vi "scan -- update freq PID .vi"() -> ()   [LabVIEW 2010]
uses:
  next chunk read-write PID -- action.ctl
  cursor window action.ctl
  find peak action.ctl
  omega map parameters.ctl
  single fit parameters.ctl
  wavepacket.ctl
  complex region.ctl
  circle corners.ctl
  lorentzian.ctl
  filter method control.ctl
panel:
  in  "file path":path=path "E:/data/Ultrasound/Experiment/ProbeTest/Probe10/YBCO_5/sweep5/June_2012/062112/61.63300K_1500_3500_001_062112.bin"
  out "Plot: All":cluster{"all rows":dbl[], "all rows":dbl[]}[](graph)
  out "Plot: complex plane - filter":cluster{dbl[], dbl[]}[](graph)=[{array[1330 elements], array[1330 elements]}, {array[1329 elements], array[1329 elements]}, {[0.0005479834959150251, 0.000546953765247259, 0.0005438686371204671, 0.000538740287125905, 0.0005315889545180808, 0.0005224428623396648, 0.0005113381060380328, 0.0004983185110130269, 0.00048343545965812373, 0.00046674768857760156, 0.0004483210567799979, 0.0004282282857626905, 0.00040654867251337085, 0.0003833677765610607, 0.00035877708231174, 0.0003328736380011912, 0.00030575967268995, 0.0002775421928119073, 0.0002483325598688017, 0.00021824605093724735, 0.00018740140372277897, 0.00015592034795637287, 0.0001239271249828129, 9.154799743686254e-05, 5.8910750942329136e-05, 2.6144189800587135e-05, -6.622371341154751e-06, -3.925961783568815e-05, -7.163874538163862e-05, -0.00010363196835519849, -0.00013511302412160458, -0.00016595767133607297, -0.00019604418026762728, -0.00022525381321073304, -0.0002534712930887757, -0.00028058525840001674, -0.0003064887027105656, -0.0003310793969598863, -0.00035426029291219646, -0.00037593990616151615, -0.0003960326771788234, -0.0004144593089764271, -0.0004311470800569493, -0.0004460301314118525, -0.00045904972643685837, -0.0004701544827384903, -0.0004793005749169064, -0.00048645190752473054, -0.0004915802575192927, -0.0004946653856460845, -0.0004956951163138507, -0.0004946653856460845, -0.0004915802575192927, -0.00048645190752473054, -0.0004793005749169064, -0.0004701544827384903, -0.00045904972643685826, -0.00044603013141185247, -0.00043114708005694924, -0.00041445930897642707, -0.00039603267717882337, -0.000375939906161516, -0.0003542602929121964, -0.00033107939695988626, -0.0003064887027105655, -0.00028058525840001685, -0.0002534712930887754, -0.00022525381321073293, -0.00019604418026762698, -0.00016595767133607288, -0.00013511302412160458, -0.00010363196835519827, -7.163874538163853e-05, -3.9259617835687814e-05, -6.622371341154649e-06, 2.6144189800587125e-05, 5.891075094232935e-05, 9.154799743686252e-05, 0.00012392712498281324, 0.00015592034795637298, 0.00018740140372277883, 0.00021824605093724757, 0.0002483325598688017, 0.0002775421928119076, 0.0003057596726899501, 0.0003328736380011915, 0.00035877708231174017, 0.0003833677765610607, 0.000406548672513371, 0.0004282282857626906, 0.0004483210567799981, 0.0004667476885776017, 0.00048343545965812373, 0.000498318511013027, 0.0005113381060380328, 0.0005224428623396649, 0.0005315889545180809, 0.000538740287125905, 0.0005438686371204671, 0.000546953765247259], [7.058823573779542e-05, 0.00010335479687953737, 0.00013599204337407076, 0.00016837117092002117, 0.0002003643938935811, 0.00023184544965998714, 0.0002626900968744556, 0.0002927766058060099, 0.00032198623874911566, 0.0003502037186271582, 0.00037731768393839946, 0.0004032211282489483, 0.000427811822498269, 0.0004509927184505791, 0.0004726723316998987, 0.0004927651027172061, 0.0005111917345148098, 0.000527879505595332, 0.0005427625569502352, 0.000555782151975241, 0.0005668869082768729, 0.000576033000455289, 0.0005831843330631132, 0.0005883126830576753, 0.0005913978111844672, 0.0005924275418522333, 0.0005913978111844672, 0.0005883126830576753, 0.0005831843330631132, 0.000576033000455289, 0.0005668869082768729, 0.000555782151975241, 0.0005427625569502351, 0.0005278795055953319, 0.0005111917345148097, 0.0004927651027172061, 0.0004726723316998987, 0.00045099271845057897, 0.0004278118224982689, 0.0004032211282489482, 0.00037731768393839946, 0.0003502037186271582, 0.00032198623874911555, 0.00029277660580600976, 0.0002626900968744555, 0.00023184544965998698, 0.00020036439389358113, 0.00016837117092002114, 0.00013599204337407065, 0.00010335479687953725, 7.058823573779526e-05, 3.7821674596053486e-05, 5.184428101520091e-06, -2.719469944443039e-05, -5.9187922417990366e-05, -9.066897818439646e-05, -0.00012151362539886495, -0.00015160013433041905, -0.00018080976727352478, -0.00020902724715156744, -0.0002361412124628087, -0.0002620446567733575, -0.0002866353510226781, -0.0003098162469749882, -0.0003314958602243079, -0.0003515886312416152, -0.0003700152630392191, -0.00038670303411974106, -0.0004015860854746444, -0.0004146056804996502, -0.00042571043680128214, -0.0004348565289796983, -0.00044200786158752237, -0.00044713621158208453, -0.00045022133970887637, -0.0004512510703766425, -0.00045022133970887637, -0.00044713621158208453, -0.00044200786158752237, -0.0004348565289796982, -0.00042571043680128214, -0.0004146056804996501, -0.0004015860854746443, -0.00038670303411974096, -0.0003700152630392189, -0.0003515886312416151, -0.0003314958602243078, -0.0003098162469749882, -0.00028663535102267787, -0.0002620446567733574, -0.00023614121246280827, -0.00020902724715156717, -0.00018080976727352478, -0.0001516001343304188, -0.00012151362539886471, -9.066897818439597e-05, -5.9187922417990095e-05, -2.719469944443035e-05, 5.184428101520362e-06, 3.782167459605353e-05]}, {array[664 elements], array[664 elements]}, {[0.00034068734716914955, 2.614418980058722e-05, 0.00036184737334241687], [0.00010448980708328159, 7.058823573779542e-05, 0.00015148623079228184]}, {[0.000403257657435818, 0.00040294817556057327, 0.00040263869368532856, 0.00040232921181008384, 0.0004020197299348392, 0.00040171024805959446, 0.00040140076618434974, 0.000401091284309105, 0.0004007818024338603, 0.0004004723205586156, 0.00040016283868337093, 0.0003998533568081262, 0.0003995438749328815, 0.0003992343930576368, 0.00039892491118239206, 0.00039861542930714734, 0.00039830594743190263, 0.00039799646555665797, 0.00039768698368141325, 0.00039737750180616853], [6.852122448113725e-05, 7.270377946499367e-05, 7.688633444885008e-05, 8.10688894327065e-05, 8.525144441656292e-05, 8.943399940041934e-05, 9.361655438427574e-05, 9.779910936813216e-05, 0.00010198166435198858, 0.00010616421933584499, 0.0001103467743197014, 0.00011452932930355783, 0.00011871188428741423, 0.00012289443927127064, 0.00012707699425512707, 0.00013125954923898347, 0.00013544210422283988, 0.0001396246592066963, 0.00014380721419055272, 0.00014798976917440912]}, {[2.614418980058722e-05, 2.875338633115941e-05, 3.13625828617316e-05, 3.397177939230379e-05, 3.658097592287598e-05, 3.9190172453448165e-05, 4.179936898402036e-05, 4.440856551459255e-05, 4.701776204516474e-05, 4.962695857573692e-05, 5.2236155106309116e-05, 5.484535163688131e-05, 5.7454548167453496e-05, 6.006374469802568e-05, 6.267294122859788e-05, 6.528213775917007e-05, 6.789133428974225e-05, 7.050053082031444e-05, 7.310972735088663e-05, 7.571892388145883e-05], [7.058823573779542e-05, 7.058823573779542e-05, 7.058823573779542e-05, 7.058823573779542e-05, 7.058823573779542e-05, 7.058823573779542e-05, 7.058823573779542e-05, 7.058823573779542e-05, 7.058823573779542e-05, 7.058823573779542e-05, 7.058823573779542e-05, 7.058823573779542e-05, 7.058823573779542e-05, 7.058823573779542e-05, 7.058823573779542e-05, 7.058823573779542e-05, 7.058823573779542e-05, 7.058823573779542e-05, 7.058823573779542e-05, 7.058823573779542e-05]}]
  out "Plot: fragment filter":cluster{dbl[], dbl[]}[](graph)
  in  "filter method":T1=enum."three"
  in  "smart filter: span 2":dbl(slide)=0.3493 min=0.0001 max=0.5 step=0.0001 scale=0.0001..0.5 scale format="%#_2g"
  out "lorentzian":T2={"Amplitude"=5.854807827548728e-05, "omega(0)"=3052.344293191275, "Gamma"=0.1436186235030105, "phase"=-1.3766021697880535, "Q"=21253.12315869183, "Norm  Ampl"=0.06539080765156977, "z (inf)"=0.4544427884804473+0.08017129776839105i, "4corners"={"z (-pi/2)"=0.09555591315300638-0.4544427884804473i, "z(inf)"=0.4544427884804473+0.08017129776839105i, "z (pi/2)"=-0.08017129776839105+0.43905817309583195i, "z center"=0.007692307692307665-0.007692307692307665i, "z(0)"=-0.43905817309583195-0.09555591315300638i, "radius"=0.4553086922616207}} {"z (inf)" format="%#9_9f"; "Q" format="%#9_9f"; "phase" format="%#9_9f"; "Gamma" format="%#9_9f"; "omega(0)" format="%#9_9f"}
  out "complex region":T4={"max re"=1.5, "min re"=-1.5, "max im"=1.5, "min im"=-1.5, "delta re"=3.0, "delta im"=3.0, "center re"=0.0, "delta  z"=3.0+3.0i, "center im"=0.0, "center z"=0.0+0.0i, "d im"=0.0, "d re"=0.0, "d z"=0.0+0.0i}
  in  "parameters: wavepacket":T5={"R"=0.5, "wave number"=24.764705882352942, "delta k"=8.0, "radii vector"=[-1.5, -1.4846153846153847, -1.4692307692307693, -1.4538461538461538, -1.4384615384615385, -1.4230769230769231, -1.4076923076923076, -1.3923076923076922, -1.376923076923077, -1.3615384615384616, -1.3461538461538463, -1.3307692307692307, -1.3153846153846154, -1.3, -1.2846153846153845, -1.2692307692307692, -1.2538461538461538, -1.2384615384615385, -1.2230769230769232, -1.2076923076923076, -1.1923076923076923, -1.176923076923077, -1.1615384615384614, -1.146153846153846, -1.1307692307692307, -1.1153846153846154, -1.1, -1.0846153846153845, -1.0692307692307692, -1.0538461538461539, -1.0384615384615383, -1.023076923076923, -1.0076923076923077, -0.9923076923076923, -0.9769230769230769, -0.9615384615384615, -0.9461538461538461, -0.9307692307692308, -0.9153846153846154, -0.8999999999999999, -0.8846153846153846, -0.8692307692307693, -0.8538461538461538, -0.8384615384615384, -0.823076923076923, -0.8076923076923077, -0.7923076923076923, -0.7769230769230768, -0.7615384615384615, -0.7461538461538462, -0.7307692307692307, -0.7153846153846153, -0.7, -0.6846153846153846, -0.6692307692307692, -0.6538461538461537, -0.6384615384615384, -0.6230769230769231, -0.6076923076923076, -0.5923076923076922, -0.5769230769230769, -0.5615384615384615, -0.5461538461538461, -0.5307692307692307, -0.5153846153846153, -0.5, -0.48461538461538467, -0.4692307692307691, -0.4538461538461538, -0.43846153846153846, -0.4230769230769229, -0.4076923076923076, -0.39230769230769225, -0.3769230769230769, -0.3615384615384616, -0.34615384615384603, -0.3307692307692307, -0.3153846153846154, -0.2999999999999998, -0.2846153846153845, -0.26923076923076916, -0.25384615384615383, -0.2384615384615385, -0.22307692307692295, -0.20769230769230762, -0.1923076923076923, -0.17692307692307674, -0.1615384615384614, -0.14615384615384608, -0.13076923076923075, -0.11538461538461542, -0.09999999999999987, -0.08461538461538454, -0.0692307692307692, -0.053846153846153655, -0.038461538461538325, -0.023076923076922995, -0.007692307692307665, 0.007692307692307665, 0.023076923076923217, 0.03846153846153855, 0.05384615384615388, 0.06923076923076943, 0.08461538461538476, 0.10000000000000009, 0.11538461538461542, 0.13076923076923075, 0.1461538461538463, 0.16153846153846163, 0.17692307692307696, 0.1923076923076925, 0.20769230769230784, 0.22307692307692317, 0.2384615384615385, 0.25384615384615383, 0.2692307692307694, 0.2846153846153847, 0.30000000000000004, 0.3153846153846156, 0.3307692307692309, 0.34615384615384626, 0.3615384615384616, 0.3769230769230769, 0.39230769230769247, 0.4076923076923078, 0.42307692307692313, 0.4384615384615387, 0.453846153846154, 0.46923076923076934, 0.48461538461538467, 0.5, 0.5153846153846153, 0.5307692307692307, 0.5461538461538464, 0.5615384615384618, 0.5769230769230771, 0.5923076923076924, 0.6076923076923078, 0.6230769230769231, 0.6384615384615384, 0.6538461538461542, 0.6692307692307695, 0.6846153846153848, 0.7000000000000002, 0.7153846153846155, 0.7307692307692308, 0.7461538461538462, 0.7615384615384615, 0.7769230769230768, 0.7923076923076926, 0.8076923076923079, 0.8230769230769233, 0.8384615384615386, 0.8538461538461539, 0.8692307692307693, 0.8846153846153846, 0.9000000000000004, 0.9153846153846157, 0.930769230769231, 0.9461538461538463, 0.9615384615384617, 0.976923076923077, 0.9923076923076923, 1.0076923076923077, 1.023076923076923, 1.0384615384615388, 1.053846153846154, 1.0692307692307694, 1.0846153846153848, 1.1, 1.1153846153846154, 1.1307692307692307, 1.1461538461538465, 1.1615384615384619, 1.1769230769230772, 1.1923076923076925, 1.2076923076923078, 1.2230769230769232, 1.2384615384615385, 1.2538461538461538, 1.2692307692307692, 1.284615384615385, 1.3000000000000003, 1.3153846153846156, 1.330769230769231, 1.3461538461538463, 1.3615384615384616, 1.376923076923077, 1.3923076923076927, 1.407692307692308, 1.4230769230769234, 1.4384615384615387, 1.453846153846154, 1.4692307692307693, 1.4846153846153847], "radial section"=[-0.0006030222864618956+0.0005497274497566944i, -3.410284436041448e-05+0.0010132859350128669i, 0.0008688436312578839+0.0009062796140498529i, 0.0015494036595505706+1.3215510930527533e-05i, 0.0013422007968163314-0.001353056497202772i, -3.874535907058629e-05-0.002336014216910577i, -0.002076341915052819-0.00195872095281468i, -0.003472679245196803+0.00014488902849802888i, -0.002816423591351656+0.0031399030948652588i, 0.0003405917207824438+0.005090163652827743i, 0.0046794137954371175+0.003989890881862977i, 0.007356579858466857-0.000678171857061158i, 0.0055683347829834275-0.00687299066125607i, -0.0012325906996523747-0.01048325607481184i, -0.009949437169656574-0.0076550907196377685i, -0.014729601858788783+0.002108083611874836i, -0.010365507233806187+0.01419604567963966i, 0.0034454547587481972+0.02040603230317615i, 0.019964962703567995+0.01382276276431399i, 0.027873832155830704-0.005429547421867458i, 0.018151205479896723-0.027676846516562437i, -0.008296145275410942-0.037540733585616916i, -0.037820319369914285-0.02346696234817867i, -0.04985099232120596+0.012337291165413702i, -0.029865810574084717+0.05094559352067978i, 0.017903766357683034+0.06526892168266896i, 0.06765069121465508+0.03740864703762122i, 0.0842552185388239-0.025403303711696697i, 0.04610531129338743-0.0885589408396967i, -0.035293068940597624-0.10723600622350836i, -0.11428695754015838-0.05589797707146281i, -0.13456531473077762+0.04806509092139521i, -0.06664576820805984+0.1454031223680393i, 0.06422370016897247+0.16648266925515984i, 0.1823776360139868+0.07811260389297386i, 0.20306847568641548-0.08425466662508742i, 0.08996045409999741-0.225526469801022i, -0.10858660194353732-0.24420085083446297i, -0.27495284597819714-0.10175011337866634i, -0.2895182954122428+0.13754625230839188i, -0.11295122460124632+0.3304910852498374i, 0.1713104538924588+0.33839299219251145i, 0.39165856773064406+0.12296258437144472i, 0.3899193919455792-0.20985861111604345i, 0.1311427674002663-0.45762196754999124i, -0.2529304170898486-0.4429220336842026i, -0.5271836745499724-0.13684990129238664i, -0.4959852129631952+0.29999399043157543i, -0.13948814023754325+0.5987933066809247i, 0.3502295017302095+0.5475052313928133i, 0.6705874359359978+0.1385571984703635i, 0.5957636952762969-0.4025326101934653i, 0.13370039949431342-0.740458204554625i, -0.45554061253945116-0.6390179277302781i, -0.8061486180679402-0.12474624762104539i, -0.6756023187520073+0.5076822072459826i, -0.1117386604048772+0.8653692868531031i, 0.5572493841777997+0.7040326776506173i, 0.9159286279708553+0.09495176570336554i, 0.7231046533352673-0.602487433797445i, 0.07488652489738247-0.9558664214239979i, -0.6416967548251327-0.7319772479362907i, -0.9835794738680782-0.052248258717673676i, -0.7302334435862515+0.6733383528082371i, -0.02790620748624336+0.9979282020574354i, 0.6961339459629277+0.7179119230644408i, 0.9983142776773428+0.0028382852950516162i, 0.6955065833561681-0.7091516142564821i, -0.021934090906148174-0.9847219696999531i, -0.7118689964171874-0.6639336929163023i, -0.9577192077429433+0.04541504527527316i, -0.624469736026339+0.7042080632498762i, 0.06670065622108534+0.918418266263491i, 0.6865382414143159+0.5786658193138536i, 0.8683998578498457-0.08503656709964526i, 0.5282466365498518-0.6596477905905617i, -0.0998616890365944-0.8096078456704449i, -0.6246864542864867-0.475003153110055i, -0.7442243314565364+0.11083453426287443i, -0.42068827479338794+0.5830851209984653i, 0.11784070416588094+0.6745362665749416i, 0.5364602224408562+0.36692385044228987i, 0.6028048562663035-0.12098210882012916i, 0.31512560287199426-0.486511644452389i, -0.12055034395435488-0.5311479424494023i, -0.4349229574901926-0.2664502671422545i, -0.46144347567335886+0.11698807368366804i, -0.22176666982095636+0.3832718526467701i, 0.11084311711439704+0.3952594517788133i, 0.3329569836082776+0.18165003673084837i, 0.33381267941878145-0.10272016173950616i, 0.14639674969272087-0.28514523769809125i, -0.09323466631364656-0.2779558419631877i, -0.24074110041966623-0.11605528095975655i, -0.22818984449402901+0.08297268678655477i, -0.09046821189732206+0.2003775369192117i, 0.07245922664442471+0.18469662010736076i, 0.16442593719966847+0.06932008368234778i, 0.16442593719966847+0.06932008368234778i, 0.07245922664442267+0.18469662010736185i, -0.0904682118973245+0.20037753691921092i, -0.2281898444940303+0.08297268678655224i, -0.24074110041966526-0.11605528095975949i, -0.09323466631364347-0.2779558419631891i, 0.1463967496927244-0.28514523769809i, 0.33381267941878145-0.10272016173950616i, 0.3329569836082776+0.18165003673084837i, 0.11084311711439261+0.39525945177881505i, -0.2217666698209607+0.38327185264676816i, -0.46144347567336064+0.11698807368366325i, -0.4349229574901901-0.2664502671422594i, -0.12055034395434933-0.5311479424494042i, 0.3151256028719998-0.4865116444523861i, 0.6028048562663035-0.12098210882012916i, 0.5364602224408562+0.36692385044228987i, 0.11784070416587385+0.6745362665749434i, -0.42068827479339543+0.5830851209984604i, -0.7442243314565383+0.11083453426286527i, -0.6246864542864821-0.47500315311006186i, -0.09986168903658582-0.8096078456704464i, 0.5282466365498591-0.6596477905905564i, 0.8683998578498457-0.08503656709964526i, 0.6865382414143159+0.5786658193138536i, 0.06670065622107231+0.9184182662634921i, -0.6244697360263467+0.7042080632498697i, -0.957719207742944+0.04541504527526296i, -0.7118689964171779-0.6639336929163127i, -0.02193409090613768-0.9847219696999534i, 0.6955065833561758-0.7091516142564748i, 0.9983142776773428+0.0028382852950516162i, 0.6961339459629277+0.7179119230644408i, -0.02790620748624336+0.9979282020574354i, -0.7302334435862515+0.6733383528082371i, -0.9835794738680771-0.05224825871769114i, -0.6416967548251248-0.7319772479362974i, 0.07488652489739264-0.955866421423997i, 0.7231046533352736-0.6024874337974371i, 0.9159286279708545+0.09495176570337203i, 0.5572493841777997+0.7040326776506173i, -0.1117386604048772+0.8653692868531031i, -0.6756023187520174+0.5076822072459677i, -0.8061486180679377-0.12474624762105674i, -0.4555406125394418-0.6390179277302841i, 0.13370039949432383-0.7404582045546224i, 0.5957636952763022-0.4025326101934566i, 0.6705874359359976+0.13855719847036346i, 0.3502295017302095+0.5475052313928133i, -0.13948814023754325+0.5987933066809247i, -0.4959852129631952+0.29999399043157543i, -0.5271836745499698-0.13684990129239397i, -0.25293041708984204-0.4429220336842057i, 0.1311427674002727-0.45762196754998885i, 0.38991939194558023-0.20985861111604046i, 0.39165856773064295+0.12296258437144741i, 0.1713104538924588+0.33839299219251145i, -0.11295122460124632+0.3304910852498374i, -0.28951829541224494+0.13754625230838535i, -0.27495284597819436-0.10175011337867199i, -0.10858660194353546-0.24420085083446344i, 0.0899604540999989-0.22552646980102106i, 0.2030684756864164-0.0842546666250844i, 0.18237763601398616+0.07811260389297513i, 0.06422370016897247+0.16648266925515984i, -0.06664576820805984+0.1454031223680393i, -0.13456531473077762+0.04806509092139521i, -0.1142869575401568-0.055897977071465065i, -0.035293068940596035-0.10723600622350866i, 0.04610531129338861-0.0885589408396959i, 0.08425521853882409-0.02540330371169545i, 0.06765069121465508+0.03740864703762122i, 0.017903766357683034+0.06526892168266896i, -0.029865810574084717+0.05094559352067978i, -0.049850992321206024+0.01233729116541259i, -0.03782031936991361-0.023466962348179375i, -0.008296145275410394-0.03754073358561696i, 0.018151205479896876-0.02767684651656224i, 0.02787383215583067-0.005429547421867246i, 0.019964962703567995+0.01382276276431399i, 0.0034454547587481972+0.02040603230317615i, -0.010365507233806187+0.01419604567963966i, -0.014729601858788783+0.002108083611874836i, -0.009949437169656303-0.00765509071963801i, -0.0012325906996522222-0.010483256074811828i, 0.005568334782983514-0.006872990661255978i, 0.007356579858466853-0.0006781718570610523i, 0.0046794137954371175+0.003989890881862977i, 0.0003405917207824438+0.005090163652827743i, -0.002816423591351656+0.0031399030948652588i, -0.0034726792451967876+0.00014488902849797876i, -0.002076341915052752-0.0019587209528147288i, -3.8745359070553e-05-0.0023360142169105715i, 0.0013422007968163269-0.0013530564972027673i, 0.0015494036595505676+1.3215510930549528e-05i, 0.0008688436312578839+0.0009062796140498529i, -3.410284436041448e-05+0.0010132859350128669i], "wave vector"=51.867078712207956, "wavepacket is"=TRUE} {"delta k" format="%#_3f"; "wave number" format="%#_3f"; "R" format="%#_3f"}
  in  "parameters: center detection":T6={"number of 2D grid points"=195, "# of points in pond"=148, "# of points in window"=1330, "decimation threshold"=1, "normalization factor"=0.0008953564021942735, "pond scale factor "=3.0, "normalized z"=array[1330 elements], "decimated z"=[0.49998884780276176+0.09267073958421544i, 0.45724397713919135+0.20178159786949873i, 0.414499106475621+0.310892456154782i, 0.4545383969166079+0.14475945108117963i, 0.4473172853578169+0.13005864280928525i, 0.4332378722238452+0.12242313425040938i, 0.4633823422941004+0.11866798510710887i, 0.4556565773470105+0.11631524095682716i, 0.45438426266266213+0.10739924486745965i, 0.4457125044076876+0.12916223117595146i, 0.43968231478121217+0.13909215522757157i, 0.43302276702957126+0.15438030761298024i, 0.4299787480691258+0.15798355285513083i, 0.4240290225857896+0.17012187215394922i, 0.4179178041950412+0.18469953518238824i, 0.4150272762225629+0.1954954379053828i, 0.4119430671246692+0.20010698040932678i, 0.40309311380722707+0.21598716517281263i, 0.39975291113676054+0.22118745274828294i, 0.39072749990711075+0.23091901070119702i, 0.38437050809060147+0.2376201906636986i, 0.3806088054849359+0.24812396854157745i, 0.3729690074855191+0.26244997379794194i, 0.3665868459360177+0.2710795782539178i, 0.3624231592276914+0.27744185192423265i, 0.35341700670302223+0.2933105004598558i, 0.3396788715122088+0.3100545603020573i, 0.3364338685487657+0.31139808773052235i, 0.31993361300627177+0.3251483203844242i, 0.3066608112921155+0.3386803444783743i, 0.2920917724235476+0.35184896238705404i, 0.2877801250908603+0.3594116842294236i, 0.27492126740652056+0.367629653693922i, 0.27163356952669393+0.37004242522727665i, 0.2567355577570752+0.38759343672442786i, 0.24613400193395804+0.4007175918608001i, 0.21551351780034478+0.41086782793871485i, 0.21148813429748808+0.4140694785202386i, 0.19500240152351508+0.42097228849382445i, 0.17188887635614356+0.43066145863110217i, 0.16691769240275425+0.43924079849257597i, 0.14489192533571155+0.45222711771481977i, 0.13379297219997238+0.4476687003611652i, 0.11289978536079444+0.449462553878249i, 0.08676269370974397+0.4570632884237847i, 0.06490166010679382+0.4625539761164954i, 0.05513306911987656+0.46036538060563476i, 0.027590625159460487+0.45698143381794054i, 0.009407927446507616+0.4573343978137928i, -0.0074079392041385295+0.4641050973122746i, -0.040399649208757465+0.46873571228297367i, -0.08510568391076283+0.45359817532308166i, -0.11768887168254957+0.4488214367231681i, -0.16704027421961382+0.42914275994131645i, -0.17340824248375034+0.41166861981952224i, -0.22757390794031+0.38643769538235045i, -0.2632093475612774+0.3539119433436539i, -0.28783941759727055+0.30902035011937207i, -0.336613455838523+0.25243652381160314i, -0.3716723343805579+0.24139662684451865i, -0.40900945655220583+0.19619952860183415i, -0.43243203500412103+0.13964144977733797i, -0.4476519041028149+0.10621198480855637i, -0.4769259032775812+0.06394771415824109i, -0.5000111521972382+0.02038909776003203i, -0.46263909427481165-0.03566853414096309i, -0.45796438931396555-0.08469903346474932i, -0.4129627378378165-0.12826404956030849i, -0.3481633259569818-0.17609919889509693i, -0.35198530121339106-0.2291485804345228i, -0.3112321032093577-0.2737902318648108i, -0.31066399229519337-0.29926189066417214i, -0.29549122551273604-0.322379605753546i, -0.2790142214825416-0.35670391010764874i, -0.2550896070552662-0.3552407803618249i, -0.23017304893314788-0.38894342352256195i, -0.20770447345548235-0.41184903963497377i, -0.17331465561037157-0.43792032246400014i, -0.12397163901539623-0.42424421881409224i, -0.09681979523477181-0.4288313605545266i, -0.06304727094357813-0.45527127700239006i, -0.026447054747576984-0.4685939185218699i, -0.027759734010551634-0.4378590116401553i, -0.013494257616258823-0.4407529318697356i, 0.007513785628294255-0.45741945176797666i, 0.017687291993971475-0.45700814379932486i, 0.03182257163497607-0.44962349705633237i, 0.05327455659123653-0.4429925775854918i, 0.07143988319779879-0.4399324083101207i, 0.08173320493909597-0.4353681709622054i, 0.09643899983786933-0.4293412599671067i, 0.11828065154584935-0.43037346306406926i, 0.13079092706433185-0.430525456069638i, 0.1526404892024-0.4368291038191696i, 0.17051632937566905-0.43422524822788333i, 0.18287043856062268-0.42204494878563076i, 0.1953102895102893-0.4228973327517883i, 0.19849790135882778-0.4127704229653055i, 0.20950924707237692-0.40582250643081463i, 0.22412639570149048-0.4044036288577729i, 0.23203444258162562-0.3954237134692515i, 0.25896089514085485-0.38900916542867475i, 0.27081188831795633-0.3873908440702499i, 0.277569470045834-0.38498930644808116i, 0.2864475651224361-0.37755865757736967i, 0.29334333688196945-0.3751103916159327i, 0.2998532248741637-0.3668730621417493i, 0.31093550954331695-0.36234944221289517i, 0.32015322738791036-0.34665204047575593i, 0.3282267130297758-0.3463425017075047i, 0.3349976004122105-0.33294873029647093i, 0.3391161130863614-0.3287674065675537i, 0.3543616648239495-0.3240848528923814i, 0.35358840907574723-0.3211329641476316i, 0.35783337669529236-0.31828682265992797i, 0.36503603577025295-0.3017022270508552i, 0.3697984174576452-0.2950045715823783i, 0.3747644290533448-0.29118393224425443i, 0.38622083903049814-0.27905818925036613i, 0.3855664704255771-0.27581265987307235i, 0.3946519479361214-0.2552894713217758i, 0.40181346102802773-0.24853116704266326i, 0.40546251026299973-0.24610844996525494i, 0.4121367410999556-0.22715899030984077i, 0.4155127852150482-0.21952255854791602i, 0.41775370189098054-0.2122210126732161i, 0.42217643249195835-0.19862093037947315i, 0.42842049171456537-0.18192696488621113i, 0.4308274182805567-0.1810916817784067i, 0.4315091988330198-0.18665466059324376i, 0.4397651947389369-0.166731604363302i, 0.4462889519346405-0.15640293393913837i, 0.4472039808848728-0.1521619030592347i, 0.4503386700789815-0.13836132721672362i, 0.45641114095521773-0.12208871944690877i, 0.45997563023411914-0.10712705758433964i, 0.4580579630837301-0.0912803637026267i, 0.4582591909330402-0.07674178707450305i, 0.4602618719812539-0.06069767445620299i, 0.4594197319898317-0.04546537144725419i, 0.45937900892871486-0.030332891533111958i, 0.459403754642652-0.014882659739605036i, 0.45976814541379296+0.0002962523607083324i, 0.46112766672467664+0.01561376716659274i, 0.4593911276216489+0.03078015731417007i, 0.4592245954535451+0.04617473574181786i, 0.45807763504011406+0.06167556269553245i, 0.45694110153953243+0.07703547304057685i], "decimated omega"=[3033.8815671938637, 3034.7185529721205, 3035.48405369871, 3036.1869760965023, 3036.8347929739775, 3037.4338225762535, 3037.989444730366, 3038.9882729772075, 3044.2215517804757, 3050.3277929190913, 3050.6904620823734, 3050.9534986946715, 3051.000234334621, 3051.311849899659, 3051.5422183510705, 3051.67020758005, 3051.7136707296513, 3051.83398547524, 3051.860644221315, 3051.916917573484, 3051.9463297800908, 3051.9749008663775, 3052.0117662128546, 3052.029700382884, 3052.0429426609962, 3052.0774205965186, 3052.1107504714714, 3052.1148399269136, 3052.1430100374982, 3052.1587610054785, 3052.1742707259937, 3052.178111411476, 3052.1857495513755, 3052.18954724731, 3052.2083267103562, 3052.215743104959, 3052.2267682960546, 3052.2304172895247, 3052.2340534267623, 3052.241287554684, 3052.2448857539307, 3052.2520449370086, 3052.2556061235377, 3052.2591551736064, 3052.2626921862015, 3052.2662172593873, 3052.2697304903163, 3052.2732319752386, 3052.276721809517, 3052.280200087633, 3052.2836669032035, 3052.287122348986, 3052.2905665168933, 3052.293999498, 3052.2974213825573, 3052.3008322599976, 3052.3042322189503, 3052.3076213472473, 3052.310999731934, 3052.314367459279, 3052.3177246147848, 3052.3210712831933, 3052.3244075484995, 3052.3277334939567, 3052.3310492020883, 3052.3343547546947, 3052.337650232863, 3052.340935716973, 3052.344211286711, 3052.347477021072, 3052.350732998372, 3052.353979296254, 3052.360443161023, 3052.3636608799056, 3052.3668692233778, 3052.3700682658377, 3052.3732580810574, 3052.3764387421916, 3052.3796103217815, 3052.3827728917654, 3052.3859265234832, 3052.3890712876846, 3052.392207254535, 3052.395334493624, 3052.3984530739704, 3052.4015630640292, 3052.4046645316994, 3052.407757544328, 3052.4108421687183, 3052.4139184711353, 3052.4169865173126, 3052.420046372457, 3052.423098101257, 3052.4261417678854, 3052.429177436009, 3052.4322051687905, 3052.4352250288975, 3052.4412413793066, 3052.4442379925113, 3052.447226978856, 3052.4502083986094, 3052.4561487770984, 3052.4591078540725, 3052.4650040757056, 3052.4679413359286, 3052.47087143874, 3052.476710398507, 3052.4796193675993, 3052.485416561429, 3052.4883048958304, 3052.494061310758, 3052.4969294985585, 3052.502646100109, 3052.505494618823, 3052.508336685511, 3052.516824687068, 3052.519641457485, 3052.5224520299894, 3052.533633330833, 3052.5364136532417, 3052.547476373588, 3052.552973252567, 3052.5557132346376, 3052.5693303953535, 3052.574739480685, 3052.58281373301, 3052.593507711284, 3052.606763758992, 3052.609400524874, 3052.612032570956, 3052.6303280789834, 3052.6406848758124, 3052.6458376007367, 3052.6611966517667, 3052.688990078296, 3052.7138798888504, 3052.760301774632, 3052.8199500741866, 3052.889949462337, 3052.963462945242, 3053.052587853033, 3053.2036812411457, 3053.353901538302, 3053.46309284956, 3053.6677854871505, 3054.021825984757, 3054.72978302167, 3056.5222677189986], "omega in window"=array[1330 elements], "z in window"=array[1330 elements], "data center"=-1.1152197238266116e-05+7.089688055188432e-05i, "inverse"=[1.221837900812892-39.02986412813202i, 1.200115507810904-39.1492602789422i, 0.8915300572458629-39.73260591525208i, 1.0166743489706092-40.2802751209584i, 0.7442630836154243-40.371271927455226i, 0.9660673250586111-41.232421494104784i, 1.1036247076236212-41.74786999505474i, 0.8971650681136023-41.889863572106464i, 0.9193864480467024-42.57357596821291i, 0.619289728909177-42.79057556636404i, 0.6073713367569147-43.192768948716285i, 0.7949959774164566-43.35074078908364i, 0.4168599321293763-43.90754625260512i, 0.7622693514390388-44.53225321272743i, 0.5545389728778318-44.79566900492336i, 0.32268785196454025-45.238970701172384i, 0.5564927377507456-45.75520521133961i, 0.3013165209143323-46.240824006000636i, 0.4198761451756224-47.01746953970865i, 0.7186537618671152-47.25256597890467i, 0.46278117693713156-47.75736491738154i, 0.973746113159675-48.455383320893446i, 0.6556263427354658-48.67940551205682i, 0.1223883728504343-49.391358622121736i, 0.5273968595776621-49.54825946756885i, 0.28123459011944646-50.0701622155107i, 0.08520315319120214-50.96630167093792i, -0.39983305032838395-51.08908998175112i, -0.3027744495973505-51.69113972894301i, -0.0050702680517821785-52.747539398720335i, -0.5974267061919301-53.518196575883636i, -0.5902286862676227-54.65458863378163i, -0.5734377556442796-55.061932074703975i, -1.2963827914881676-55.855902566307876i, -1.557259570968706-55.94244453354828i, -1.783391090850398-56.539103827431695i, -1.6926544573059237-57.57041809061103i, -1.0997648103320967-57.90652740864441i, -0.709875450194623-58.88586409838409i, -1.031052910920114-59.47750545766915i, -2.0239047151952625-59.66700036328392i, -2.415358861437403-61.70243999579684i, -2.8551768497774916-61.718202104091475i, -3.160868434730999-62.77653037430503i, -3.7937509645227743-63.91637358644423i], "linear "=[-42.68416750837511+3.5212848792575673i, -42.81128455615866+3.5613048660496154i, -43.404626269869944+3.977425100230206i, -44.01849607621949+3.9160748835933363i, -44.080337135669666+4.225351780557317i, -45.04900760223429+4.101614570113604i, -45.62947029118234+4.022326546499945i, -45.75590881622412+4.266727839251642i, -46.503913357017666+4.336152156437181i, -46.699253288338745+4.692851086779986i, -47.13584401825904+4.760918685298091i, -47.33366314304101+4.578120797168566i, -47.888561990191945+5.066387410485337i, -48.61653674136788+4.775590640478541i, -48.87510079099175+5.038005625111108i, -49.326362021739385+5.351338039848642i, -49.92086250113941+5.167288039372887i, -50.415037276031505+5.511830523750367i, -51.27749395972759+5.489013804507114i, -51.5745694351289+5.19566797906467i, -52.08954719504087+5.543595989185196i, -52.920074130448825+5.082452987166939i, -53.12059745030248+5.459751288023236i, -53.82330085483412+6.138262198906403i, -54.04972437577889+5.71845993757443i, -54.584668007343915+6.058150170254591i, -55.53423907421064+6.39447148827731i, -55.60160002174818+6.939774795120276i, -56.270875515211806+6.916473833297858i, -57.46268184571373+6.736777409358649i, -58.22125174966319+7.487742474159611i, -59.46043076741757+7.635531748451848i, -59.906564735639066+7.673023478089221i, -60.67265194722145+8.56946845595019i, -60.73121877101723+8.865567472756844i, -61.350359116372935+9.193670666266078i, -62.48648802732039+9.236047003108121i, -62.9339048731064+8.636075771287427i, -64.05436972830942+8.34538196978159i, -64.65502580752391+8.776358364291445i, -64.72552232701196+9.884104467217032i, -66.88969156514364+10.589385394091076i, -66.8466313671+11.070762170145418i, -67.95790230716948+11.548779515997872i, -69.11318079788546+12.394462186573897i], "omega around"=[3053.6194141237424, 3053.622573931677, 3053.625742701614, 3053.628920504767, 3053.6321074129446, 3053.6353034985545, 3053.638508834613, 3053.641723494751, 3053.644947553222, 3053.6481810849077, 3053.6514241653276, 3053.654676870645, 3053.6579392776757, 3053.6612114638956, 3053.664493507448, 3053.6677854871505, 3053.671087482506, 3053.6743995737097, 3053.677721841655, 3053.6810543679453, 3053.6843972349006, 3053.687750525567, 3053.6911143237244, 3053.6944887138966, 3053.6978737813592, 3053.7012696121506, 3053.7046762930795, 3053.708093911733, 3053.7115225564908, 3053.7149623165296, 3053.7184132818375, 3053.72187554322, 3053.725349192312, 3053.7288343215887, 3053.7323310243746, 3053.735839394855, 3053.7393595280846, 3053.7428915200026, 3053.746435467439, 3053.7499914681284, 3053.7535596207213, 3053.7571400247944, 3053.760732780863, 3053.7643379903916, 3053.7679557558095], "phase around center"=array[1330 elements], "fit for phase around senter "=[], "three points"={[3052.2724838795234, 3052.344293191275, 3052.4161025030267], [1.6399532953988492, 3.2107496221937457, 4.781545948988642]}, "max omega"=3056.5222677189986, "min omega"=3033.8815671938637}
  in  "parameters: omega map":T7={"map method"=enum."around center", "2:window factor"=3, "left"=673.0175169785733, "right"=676.1124780713627, "omega"=3052.344293191275, "gamma"=0.1436186235030105, "theta0"=3.2107496221937457, "use points"=enum."all in window", "z(inf) method"=enum."histogram"}
  out "Array":T8(array[cluster])
  out "Ring Text.Text":string
  in  "freq PID OUT":T9(ring)
  out "PID freq":dbl[](array[numeric])
  out "complex plane norm":dbl=0.0005218393061144379
  out "complex plane center":cdb=2.614418980058722e-05+7.058823573779542e-05i
  in  "smart filter: span":dbl(slide)=0.3493 min=0.0001 max=0.5 step=0.0001 scale=0.0001..0.5 scale format="%#_2g"
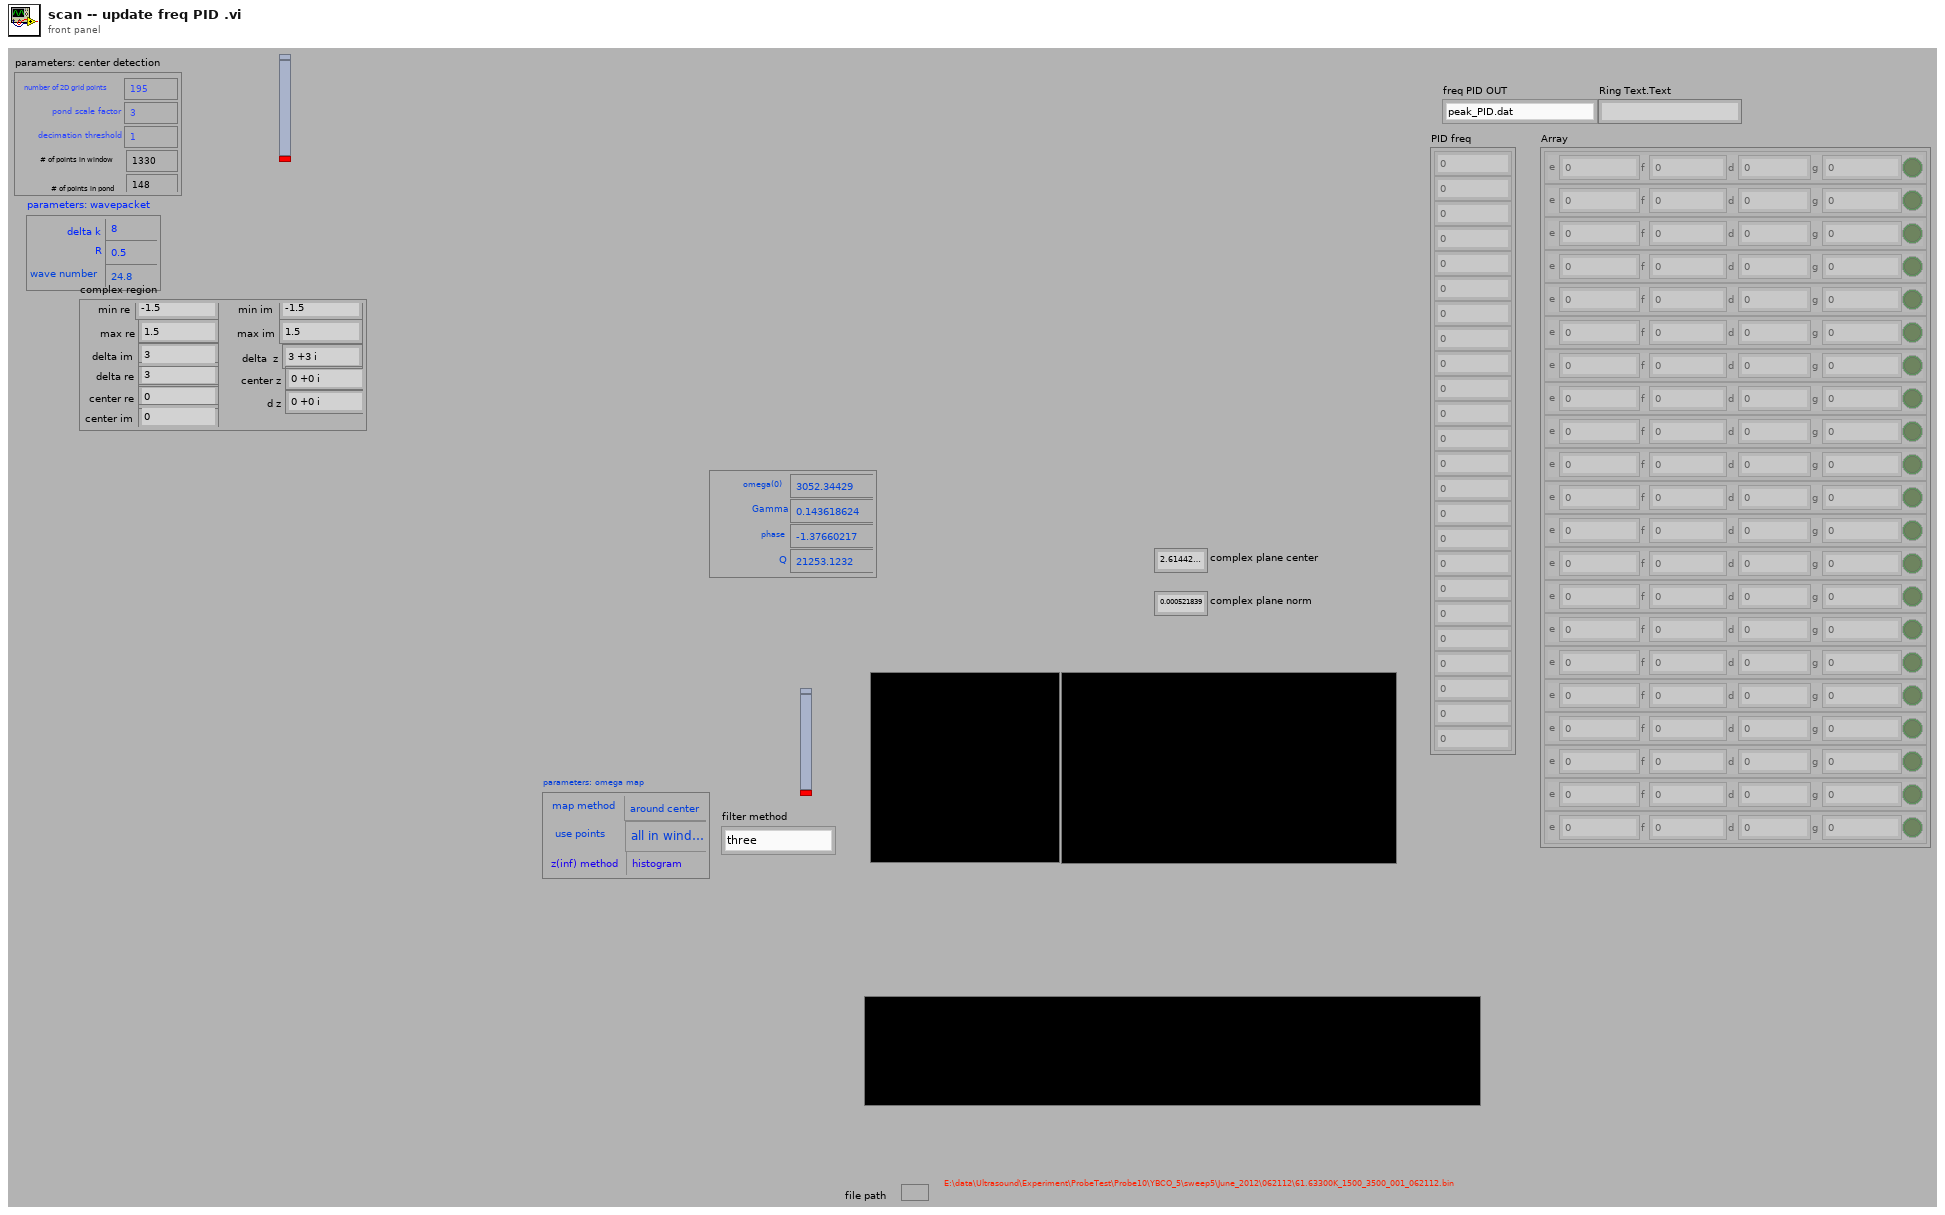
[diagram p1: front panel]
types:
  T1 = typedef "filter method control.ctl" = enum16{"four", "five", "one", "two", "three", "zero", "minus one", "minus two"}
  T2 = typedef "lorentzian.ctl" = cluster{"Amplitude":dbl, "omega(0)":dbl, "Gamma":dbl, "phase":dbl, "Q":dbl, "Norm  Ampl":dbl, "z (inf)":cdb, "4corners":T3}
  T3 = typedef "circle corners.ctl" = cluster{"z (-pi/2)":cdb, "z(inf)":cdb, "z (pi/2)":cdb, "z center":cdb, "z(0)":cdb, "radius":dbl}
  T4 = typedef "complex region.ctl" = cluster{"max re":dbl, "min re":dbl, "max im":dbl, "min im":dbl, "delta re":dbl, "delta im":dbl, "center re":dbl, "delta  z":cdb, "center im":dbl, "center z":cdb, "d im":dbl, "d re":dbl, "d z":cdb}
  T5 = typedef "wavepacket.ctl" = cluster{"R":dbl, "wave number":dbl, "delta k":dbl, "radii vector":dbl[], "radial section":cdb[], "wave vector":dbl, "wavepacket is":bool}
  T6 = typedef "single fit parameters.ctl" = cluster{"number of 2D grid points":i32, "# of points in pond":i32, "# of points in window":i32, "decimation threshold":i32, "normalization factor":dbl, "pond scale factor ":dbl, "normalized z":cdb[], "decimated z":cdb[], "decimated omega":dbl[], "omega in window":dbl[], "z in window":cdb[], "data center":cdb, "inverse":cdb[], "linear ":cdb[], "omega around":dbl[], "phase around center":dbl[], "fit for phase around senter ":dbl[], "three points":cluster{dbl[], dbl[]}, "max omega":dbl, "min omega":dbl}
  T7 = typedef "omega map parameters.ctl" = cluster{"map method":enum16{"simple", "less trivial", "around center", "geometry"}, "2:window factor":i32, "left":dbl, "right":dbl, "omega":dbl, "gamma":dbl, "theta0":dbl, "use points":enum16{"all in window", "decimated"}, "z(inf) method":enum16{"median", "method 2", "histogram"}}
  T8 = cluster{"found":dbl, "found":bool, "exp":dbl, "gamma":dbl, "delta":dbl}[]
  T9 = enum16{"peak_PID.dat", "peak_PID_scratch.dat", "one"}
  T10 = typedef "next chunk read-write PID -- action.ctl" = enum16{"read", "interpolate", "append", "write", ""}
  T11 = cluster{"found":dbl, "found":bool, "exp":dbl, "gamma":dbl, "delta":dbl}
  T12 = typedef "find peak action.ctl" = enum16{"empty", "-find center", "-mapping", "fit", "-shake it one", "bbb", "-update pond", "move z(center)", "move z(inf)", "update pond", "fancy fit one", "fragment window moves", "-shake it two", "fancy fit two"}
  T13 = typedef "cursor window action.ctl" = enum16{"balance", "h. offset change", "cursor moves", "change center", "change window", "init", "check", "reset", "set y to middle", "idle", "-write all Y", "-write left.X", "-write center.X", "-write right.X", "-write all X", "-change center", "-change window", "-change skew", "-read cursor 2", "-read cursor 1", "-read cursor 0", "-read all cursors", "-reset", "-read plot scale", "-set y to middle", "-Q: center.Y is visible", "-Q: window is visible", "-parse center.Y", "-right left from center", "-left move", "-right move", "-set center.Y", "-empty", "-set cursors to default", "-check", "-write center.Y", "-copy cursor 1", "-copy cursor 0", "-copy cursor 2", "move right", "move left", "shrink", "broaden", "skew up", "skew down", "-write plot scale", "zoom X", "change cen&win"}
  T14 = typedef "cursor winow.ctl" = cluster{"left":dbl, "right ":dbl, "center":dbl, "window":dbl, "cursors":i32[], "relative":i32, "absolute":i32, "fixed vertical offset":dbl, "vertical offset":dbl, "skew":dbl, "default window frac":dbl, "kind":enum16{"symmetric", "skewed", "fancy"}, "skew.left":dbl, "skew.right":dbl, "Plot ref":refnum<vi>, "wing order":enum16{"forw", "back"}}
  T15 = typedef "tale of three indices -- int -- control.ctl" = cluster{"left":i32, "center":i32, "right":i32, "right most":i32, "left most":i32, "window":i32, "max win factor":i32, "max win":i32, "min win":i32}
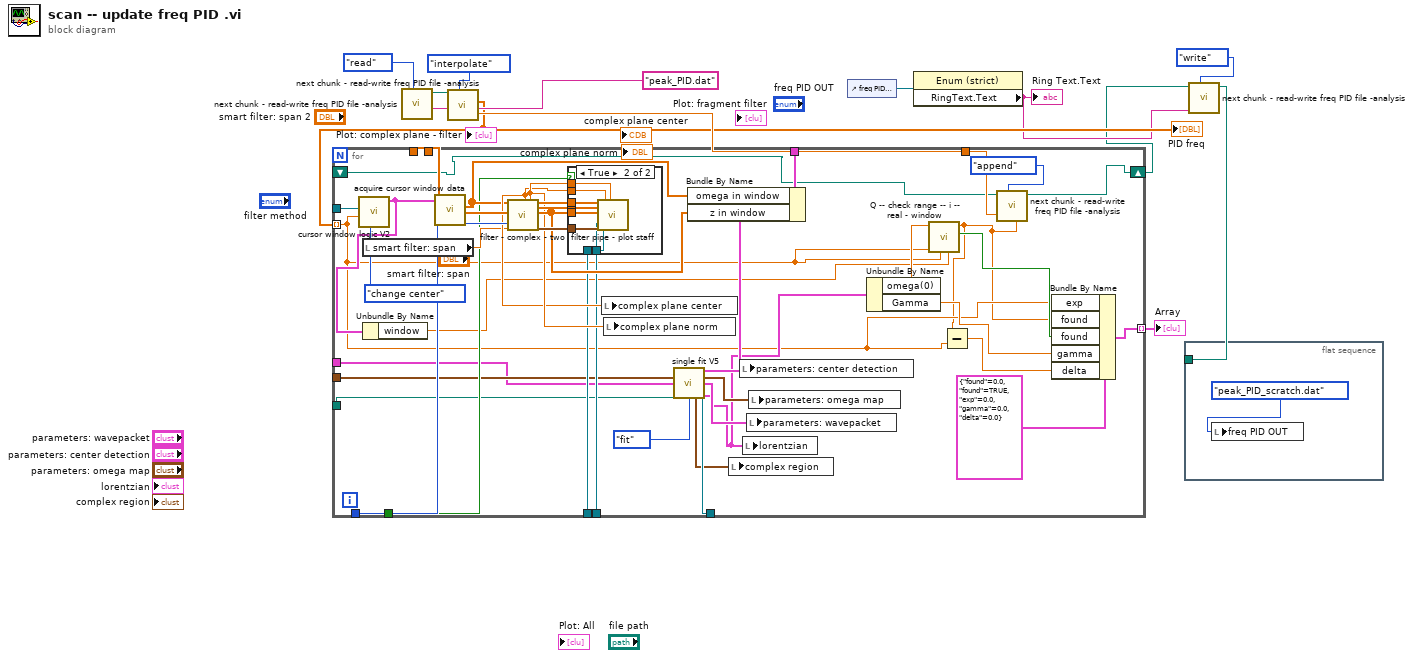
[diagram p0: block diagram]
diagram:
  n1 = call "next chunk - read-write freq PID file -analysis.vi"("PID action"=next_chunk_read-write_PID_--_action."read", "freq PID file IN"="peak_PID.dat") -> ("sweep folder path out"=w26:path, "sweep folder path"=w4:path)  [unwired: 5 in, 3 out]
  n2 = call "next chunk - read-write freq PID file -analysis.vi"("PID action"=next_chunk_read-write_PID_--_action."interpolate", "sweep folder path"=w26) -> ("PID freq"=w8:dbl[], "temperature"=w10:dbl)  [unwired: 5 in, 3 out]
  "PID freq" <- w8
  n3 = for {
    tunnel: w8 -> [w29] mode=indexing
    tunnel: [w69] -> w22
    tunnel: [w67] -> w12
    tunnel: [w66] -> w11
    tunnel: [w60] -> w21
    tunnel: [w57] -> w20
    tunnel: [w56] -> w19
    tunnel: [w53] -> w18
    tunnel: [w52] -> w17
    tunnel: [w50] -> w16
    tunnel: [w49] -> w15
    tunnel: [w47] -> w14
    tunnel: [w42] -> w13
    tunnel: w10 -> [w38]
    tunnel: [w35] -> w1 mode=indexing
    shift-right: [w33] -> w3
    shift-left: [w34] -> w5
    n4 = call "cursor window logic V2.vi"("cursor window action"=cursor_window_action."change center", "center"=w29, "cursor window in"=w69) -> ("cursor window out"=w32:T14)  [unwired: 7 in, 1 out]
    n5 = local read "smart filter: span"() -> (w54:dbl)
    n6 = Unbundle By Name(w32) -> ("window"=w31:dbl)
    n7 = call "acquire cursor window data.vi"("z in"=w66, "omega in"=w67, "cursor window"=w32) -> ("z out"=w62:cdb[], "omega  out"=w55:dbl[])  [unwired: 7 in]
    n8 = call "filter - complex - two.vi"("omega  in"=w55, "z in"=w62, "span"=w54, "filter method"=w60) -> ("center"=w58:cdb, "norm"=w59:dbl, "omega out"=w63:dbl[], "z in out"=w64:cdb[], "z out"=w61:cdb[], "tale of three"=w65:T15)  [unwired: 10 in]
    n9 = case shown="True" w53 {
      tunnel: w65 -> [_ w77]
      tunnel: w64 -> [_ w76]
      tunnel: w58 -> [_ w75]
      tunnel: w59 -> [_ w74]
      tunnel: w63 -> [_ w73]
      tunnel: w61 -> [_ w72]
      tunnel: w57 -> [_ w71]
      tunnel: w56 -> [_ w70]
      frame False {
      }
      frame True {
        n10 = call "filter pipe - plot staff.vi"("omega  in"=w73, "zin"=w76, "z out"=w72, "tale of three indices -- int -- control"=w77, "center"=w75, "Plot: complex plane - filter"=w70, "norm"=w74, "Plot: fragment"=w71) -> ()  [unwired: 12 in]
      }
    }
    n11 = local write "complex plane center"(w58) -> ()
    n12 = local write "complex plane norm"(w59) -> ()
    n13 = Bundle By Name(cluster=w52, "omega in window"=w55, "z in window"=w61) -> (w51:cluster{})
    n14 = call "single fit V5.vi"("single fit parameters"=w51, "find fit action"=find_peak_action."fit", "cursor bracket: fragment  ref"=w47, "omega map parameters"=w50, "parameters: wavepacket"=w49, "main VI path"=w42) -> ("single fit parameters out"=w46:T6, "omega map parameters out"=w45:T7, "parameters: wavepacket  out"=w44:T5, "complex region out"=w43:T4, "lorentzian out"=w41:T2)  [unwired: 5 in]
    n15 = local write "complex region"(w43) -> ()
    n16 = local write "parameters: center detection"(w46) -> ()
    n17 = local write "lorentzian"(w41) -> ()
    n18 = local write "parameters: wavepacket"(w44) -> ()
    n19 = local write "parameters: omega map"(w45) -> ()
    n20 = Unbundle By Name(w41) -> ("omega(0)"=w40:dbl, "Gamma"=w30:dbl)
    n21 = call "Q -- check range -- i -- real - window.vi"("window"=w31, "center"=w29, "default"=w29, "number"=w40) -> ("in range?"=w36:bool, "number in range"=w28:dbl)  [unwired: 5 in, 1 out]
    n22 = Subtract(x=w28, y=w29) -> (x-y=w27:dbl)
    n23 = call "next chunk - read-write freq PID file -analysis.vi"("frequency"=w28, "temperature"=w38, "PID action"=next_chunk_read-write_PID_--_action."append", "sweep folder path"=w34) -> ("sweep folder path out"=w33:path)  [unwired: 4 in, 3 out]
    n24 = Bundle By Name(cluster=T11 {"found"=0.0, "found"=TRUE, "exp"=0.0, "gamma"=0.0, "delta"=0.0}, "exp"=w29, "found"=w28, "found"=w36, "gamma"=w30, "delta"=w27) -> (w35:T11)
  }
  "Array" <- w1
  n25 = control-ref of="freq PID OUT"() -> (w9:refnum<vi>)
  n26 = property class="Enum (strict)"(reference=w9) -> ("RingText.Text"=w7:string)  [unwired: 1 in, 2 out]
  "Ring Text.Text" <- w7
  n27 = flat-sequence {
    tunnel: w2 -> [_]
    frame #0 {
      n28 = local write "freq PID OUT"(T9."peak_PID_scratch.dat" ("filter method")) -> ()
    }
  }
  n29 = call "next chunk - read-write freq PID file -analysis.vi"("PID action"=next_chunk_read-write_PID_--_action."write", "freq PID file OUT"=w7, "sweep folder path"=w3) -> ("sweep folder path out"=w2:path)  [unwired: 5 in, 3 out]
